vi "set acquisition configuration.vi"(8 "error in (no error)":errorcluster, 11 "Channel in":refnum<class "Channel.lvclass">) -> (0 "error out":errorcluster, 3 "Channel out":refnum<class "Channel.lvclass">)   [LabVIEW 2018, in "Channel.lvclass"]
uses:
  Channel.lvclass
  Channel.lvclass/Channel.ctl
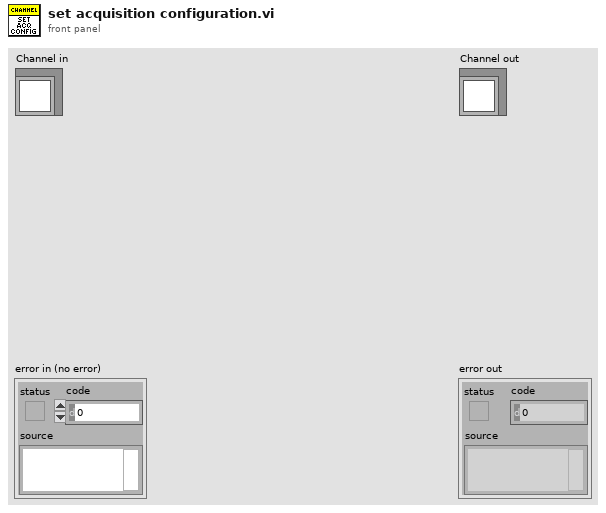
[diagram p1: front panel]
types:
  T1 = cluster{"suffix":string, "#CYCLES":u32, "#SEQS":u32, "WAVEPLATE_POS":u16, "Waveplate positions":u8[]}
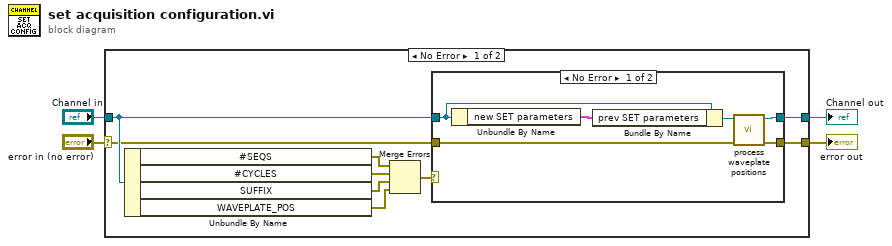
[diagram p0: block diagram]
diagram:
  n1 = case shown="No Error" "error in (no error)" {
    selector: "error in (no error)" -> [w6 w23]
    tunnel: [w5 w23] -> w3
    tunnel: [w7 w22] -> w1
    tunnel: "Channel in" -> [w8 w22]
    frame No Error {
      n2 = Unbundle By Name(w8) -> ("#SEQS"=w13:errorcluster, "#CYCLES"=w12:errorcluster, "SUFFIX"=w11:errorcluster, "WAVEPLATE_POS"=w10:errorcluster)
      n3 = Merge Errors(w13, w12, w11, w10) -> (w9:errorcluster)
      n4 = case shown="No Error" w9 {
        tunnel: w8 -> [w14 w21]
        tunnel: [w17 w21] -> w7
        tunnel: w6 -> [w16 w20]
        tunnel: [w15 w20] -> w5
        frame No Error {
          n5 = Unbundle By Name(w14) -> ("new SET parameters"=w19:T1)
          n6 = Bundle By Name(cluster=w14, "prev SET parameters"=w19) -> (w18:refnum<class "Channel.lvclass">)
          n7 = call "process waveplate positions.vi"("error in (no error)"=w16, "Channel in"=w18) -> ("error out"=w15:errorcluster, "Channel out"=w17:refnum<class "Channel.lvclass">)  [unwired: 8 in]
        }
        frame Error {
        }
      }
    }
    frame Error {
    }
  }
  "error out" <- w3
  "Channel out" <- w1
